vi "From JSON.vi"(8 "error in (no error)":errorcluster, 11 "Framework Configuration in":refnum<class "Framework Configuration.lvclass">) -> (0 "error out":errorcluster, 3 "Framework Configuration out":refnum<class "Framework Configuration.lvclass">)   [LabVIEW 2017, in "Data Sharing Framework Core.lvlib" / "Data Sharing Framework Engine.lvlib" / "Framework Configuration.lvclass"]
uses:
  Framework Configuration.lvclass
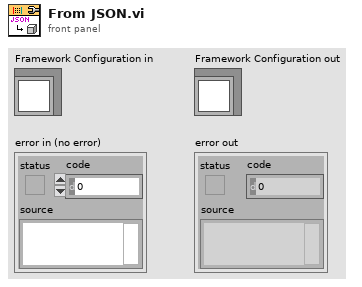
[diagram p1: front panel]
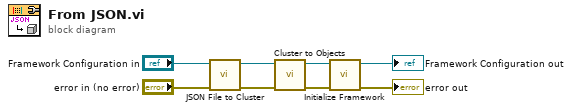
[diagram p0: block diagram]
diagram:
  n1 = call "JSON File to Cluster.vi"("error in (no error)"="error in (no error)", "Framework Configuration in"="Framework Configuration in") -> ("error out"=w6:errorcluster, "Framework Configuration out"=w7:refnum<class "Framework Configuration.lvclass">)  [unwired: 8 in]
  n2 = call "Cluster to Objects.vi"("error in (no error)"=w6, "Framework Configuration in"=w7) -> ("error out"=w3:errorcluster, "Framework Configuration out"=w4:refnum<class "Framework Configuration.lvclass">)  [unwired: 8 in]
  n3 = call-dynamic "Initialize Framework.vi"("error in (no error)"=w3, "Framework Configuration in"=w4) -> ("error out"=→"error out":errorcluster, "Framework Configuration out"=→"Framework Configuration out":refnum<class "Framework Configuration.lvclass">)  [unwired: 8 in]
